vi "B-Lockin_time.vi"(7 "remote lockin address":string, 8 "error in (no error)":errorcluster, 9 "notifier":refnum<notifier>, 10 "Experiment Description":string="cool down\n\n", 11 "Experiment Folder":string="cooldown") -> (0 "error out":errorcluster)   [LabVIEW 2016, in "Transport.lvclass"]
uses:
  Transport.lvclass
  SweepControl/SweepControl.lvclass
  <userlib>/LevyLab/Levylab Instruments/Instrument Types/Cryostat/Instrument.Cryostat.lvclass
  <userlib>/LevyLab/LV to ITX/LVtoITX.lvclass
  Control Experiment/Control Experiment.lvclass
panel:
  in  "Tab Control":T1(tab)
  in  "milliseconds to wait":u32=1000
  in  "stop":bool
  out "X Channels":dbl[](array[numeric]) format="%#_6p"
  out "Y Channels":dbl[](array[numeric]) format="%#_6p"
  in  "append to existing file?\n(new file:F)":bool
  in  "Number of Channels to Save":i32=16
  in  "V2":i32=1 min=1
  in  "Current":i32=1 min=1
  in  "V1":i32=1 min=1
  out "Y":cluster{"Y":dbl[], "Y":dbl[]}[](graph)
  out "X":cluster{"Y":dbl[], "Y":dbl[]}[](graph)
  out "R vs time":cluster{"Y":dbl[], "Y":dbl[]}[](graph)
  out "Temperature vs time":cluster{"Y":dbl[], "Y":dbl[]}[](graph)
  out "R vs T":cluster{"Y":dbl[], "Y":dbl[]}[](graph)
  out "B vs Time":cluster{"Y":dbl[], "Y":dbl[]}[](graph)
  out "R vs B":cluster{"Y":dbl[], "Y":dbl[]}[](graph)
  in  "SweepControl.lvclass":refnum<class "SweepControl.lvclass">
  # "If V1 /= V2:\nR = (V1-V2)/I\nIf V1 = V2:\nR = V1/I"
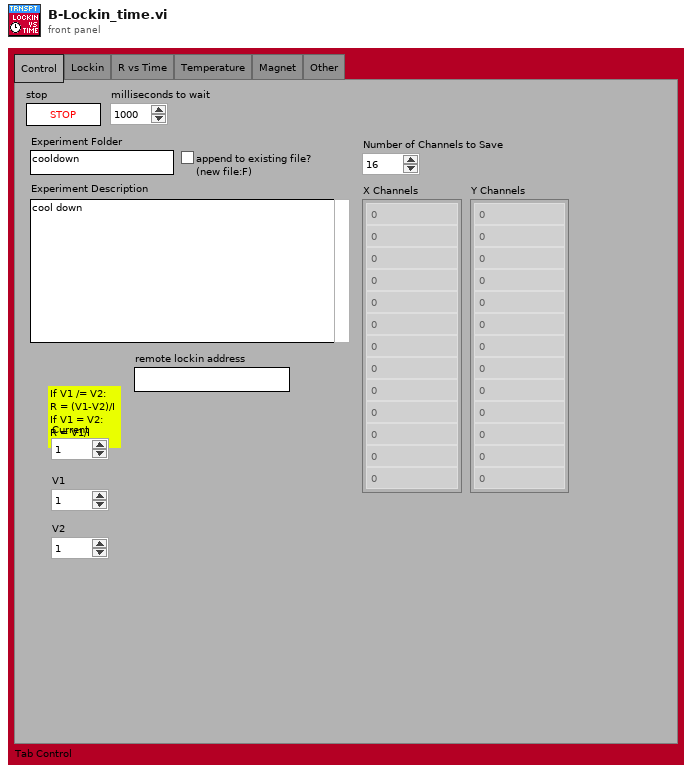
[diagram p1: front panel]
types:
  T1 = enum32{"Control", "Lockin", "R vs Time", "Temperature", "Magnet", "Other"}
  T2 = typedef "AO-cluster.ctl" = cluster{"AO amp (V)":T3, "AO DC (V)":T4, "AO f (Hz)":T5, "AO phi (°)":T6, "function":T7, "I+":bool[]}
  T3 = typedef "AO_Amp-array.ctl" = dbl[]
  T4 = typedef "AO_DC-array.ctl" = dbl[]
  T5 = typedef "AO_f-array.ctl" = dbl[]
  T6 = typedef "AO_phi-array.ctl" = dbl[]
  T7 = typedef "Function-array.ctl" = T8[]
  T8 = typedef "Function-enum.ctl" = enum16{"Sine", "Triangle", "Square", "Sawtooth"}
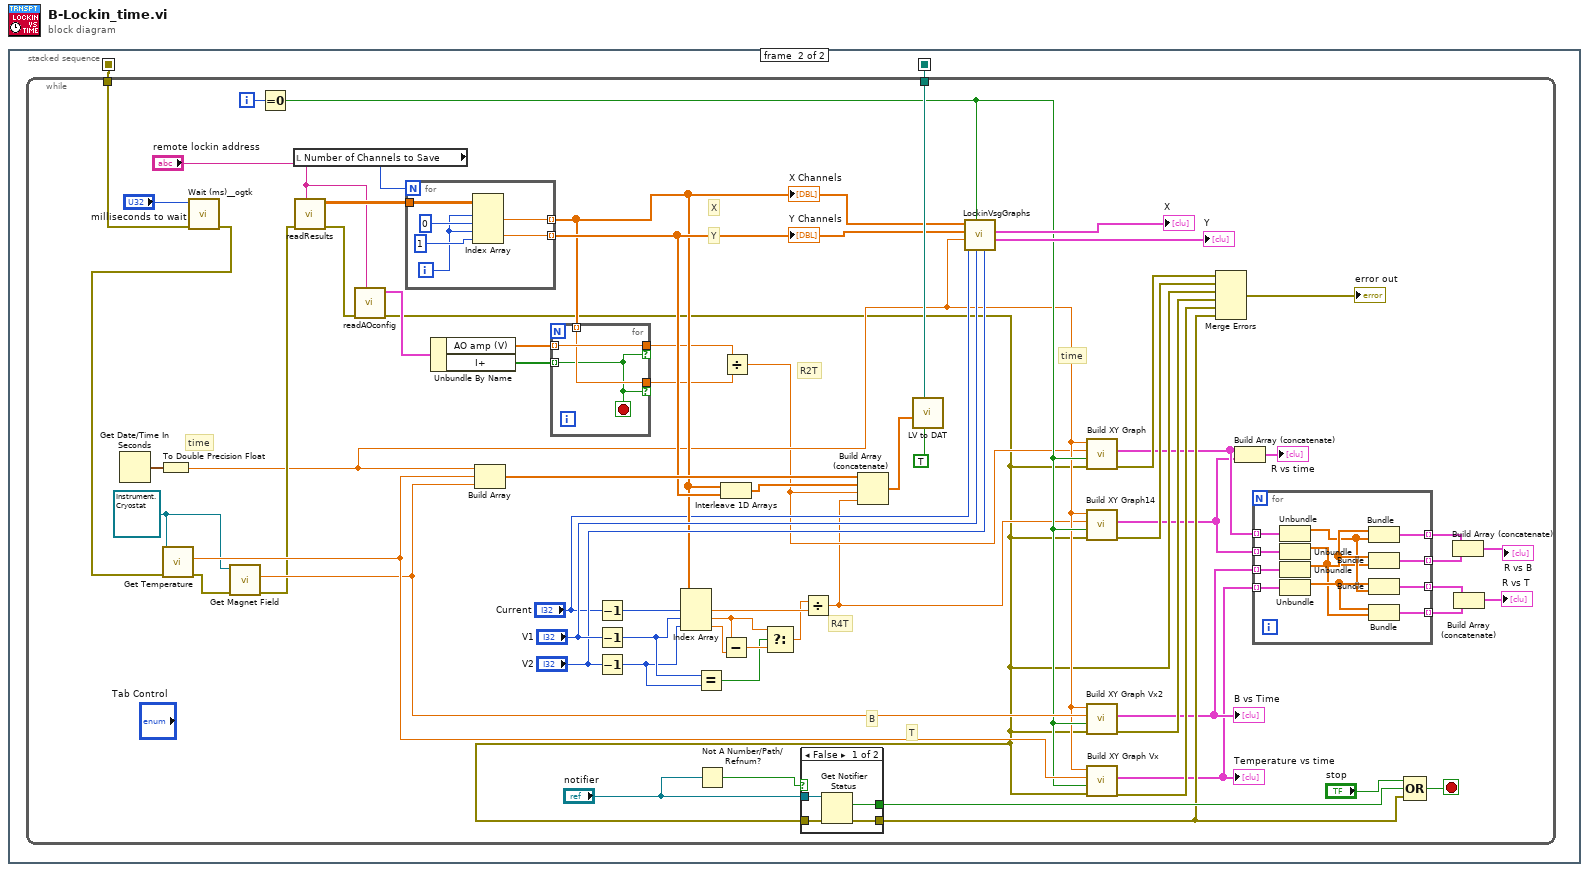
[diagram p0: block diagram]
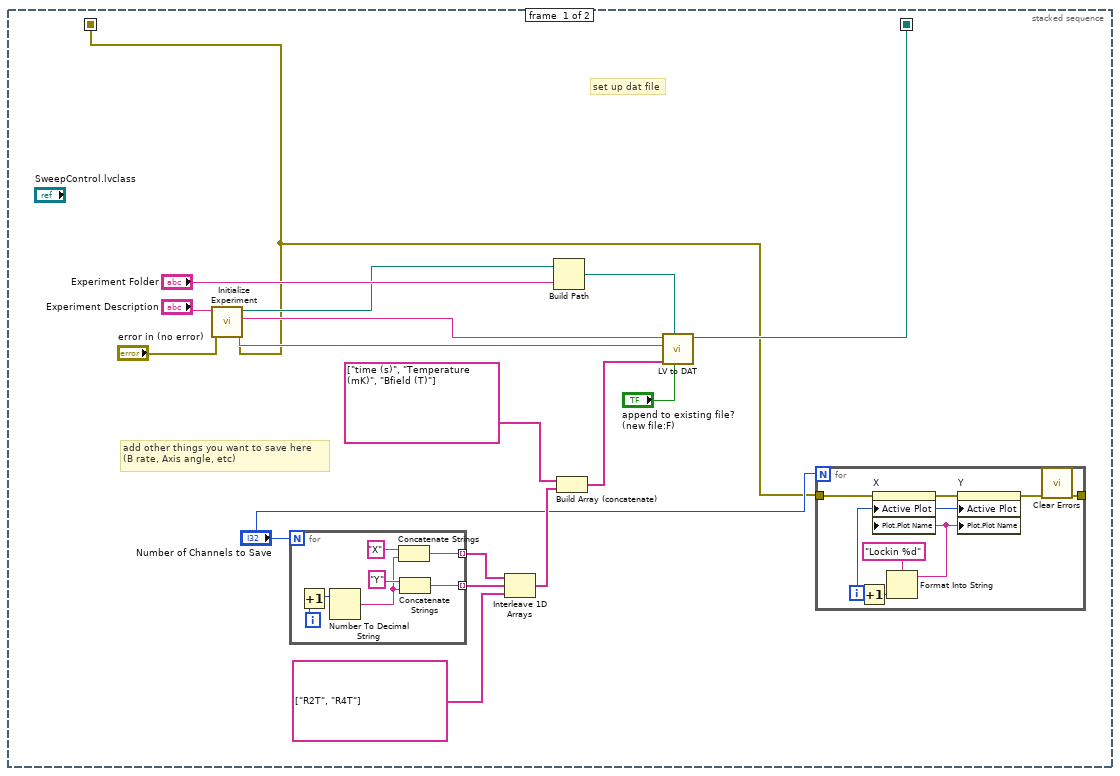
[diagram p2: hidden frame]
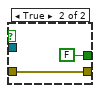
[diagram p3: hidden frame]
diagram:
  n1 = stacked-sequence {
    seq-local: [w3 _] -> [_ w34]
    seq-local: [w1 _] -> [_ w33]
    frame #0 {
      # "add other things you want to save here\n(B rate, Axis angle, etc)"
      # "set up dat file"
      n2 = call "Initialize Experiment.vi"("error in (no error)"="error in (no error)", "Experiment Comments"="Experiment Description") -> ("error out"=w1:errorcluster, "Comments"=w9:string, "device"=w8:string, "path"=w7:path)  [unwired: 6 in]
      n3 = for {
        N: "Number of Channels to Save" -> [_]
        tunnel: [w28] -> w13 mode=indexing
        tunnel: [w27] -> w12 mode=indexing
        i -> [w30]
        n4 = Increment(x=w30) -> (x+1=w26:i32)
        n5 = Number To Decimal String(number=w26) -> (decimal integer string=w29:string)  [unwired: 1 in]
        n6 = Concatenate Strings("X" ("wavenames"), w29) -> (w28:string)
        n7 = Concatenate Strings("Y" ("wavenames"), w29) -> (w27:string)
      }
      n8 = Interleave 1D Arrays(w13, w12, string[] ["R2T", "R4T"] ("wavenames (.Vx, etc)")) -> (w11:string[])
      n9 = Build Path(base path=w7, name or relative path="Experiment Folder") -> (appended path=w15:path)
      n10 = Build Array (concatenate)(string[] ["time (s)", "Temperature (mK)", "Bfield (T)"] ("wavenames (.Vx, etc)"), w11) -> (w14:string[])
      n11 = call <userlib>:"LV to DAT.vi"("append to file? (new file:F)"="append to existing file?\n(new file:F)", "path"=w15, "wavenames (.Vx, etc)"=w14, "Comments"=w9, "filename"=w8) -> ("new file path"=w3:path)  [unwired: 6 in]
      n12 = for {
        N: "Number of Channels to Save" -> [_]
        tunnel: [w24] -> _
        tunnel: w1 -> [w23]
        i -> [w21]
        n13 = Increment(x=w21) -> (x+1=w18:i32)
        n14 = Format Into String(format string="Lockin %d", w18) -> (resulting string=w22:string)  [unwired: 2 in, 1 out]
        n15 = property on="X" class="XYGraph (strict)"(error in=w23, "Active Plot"=w21, "Plot.Plot Name"=w22) -> (error out=w20:errorcluster)  [unwired: 1 in, 1 out]
        n16 = property on="Y" class="XYGraph (strict)"(error in=w20, "Active Plot"=w21, "Plot.Plot Name"=w22) -> (error out=w19:errorcluster)  [unwired: 1 in, 1 out]
        n17 = call <vilib>:"Clear Errors.vi"("error in (no error)"=w19) -> ("error out"=w24:errorcluster)  [unwired: 5 in, 1 out]
      }
    }
    frame #1 {
      n18 = while {
        tunnel: w34 -> [w100]
        tunnel: w33 -> [w78]
        i -> [w101]
        stop <- w70 stop-if-true
        w63 = refnum<class "Instrument.Cryostat.lvclass"> refnum ("Instrument.Cryostat in")
        # "R2T"
        # "R4T"
        # "T"
        # "B"
        # "time"
        # "Y"
        # "X"
        # "time"
        n19 = Get Date/Time In Seconds() -> (seconds since 1Jan1904=w98:timestamp)
        n20 = To Double Precision Float(number=w98) -> (double precision float=w50:dbl)
        n21 = call <userlib>:"Wait (ms)__ogtk.vi"("error in (no error)"=w78, "milliseconds to wait"="milliseconds to wait") -> ("error out"=w52:errorcluster)  [unwired: 8 in, 1 out]
        n22 = call-dynamic "Get Temperature.vi"("error in (no error)"=w52, "Instrument.Cryostat in"=w63) -> ("error out"=w65:errorcluster, "Temperature (K)"=w84:dbl)  [unwired: 6 in, 2 out]
        n23 = call-dynamic "Get Magnet Field.vi"("error in (no error)"=w65, "Instrument.Cryostat in"=w63) -> ("error out"=w64:errorcluster, "B Field (T)"=w79:dbl)  [unwired: 6 in, 2 out]
        n24 = Equal To 0?(x=w101) -> (x = 0?=w54:bool)
        n25 = local read "Number of Channels to Save"() -> (w93:i32)
        n26 = call <userlib>:"readResults.vi"("address"="remote lockin address", "error in (no error)"=w64) -> ("error out"=w62:errorcluster, "Results"=w99:dbl[][])  [unwired: 7 in, 1 out]
        n27 = call <userlib>:"readAOconfig.vi"("address"="remote lockin address", "error in (no error)"=w62) -> ("error out"=w46:errorcluster, "AOconfig"=w53:T2)  [unwired: 8 in]
        n28 = for {
          N: w93 -> [_]
          tunnel: w99 -> [w126]
          tunnel: [w124] -> w59 mode=indexing
          tunnel: [w125] -> w66 mode=indexing
          i -> [w123]
          n29 = Index Array(array=w126, index (row) #1=w123, index (col) #1=0 ("disabled index (col)"), index (row) #2=w123, index (col) #2=1 ("disabled index (col)")) -> (element #1=w124:dbl, element #2=w125:dbl)
        }
        "X Channels" <- w59
        "Y Channels" <- w66
        n30 = Unbundle By Name(w53) -> ("AO amp (V)"=w61:T3, "I+"=w60:bool[])
        n31 = Build Array(w50, w84, w79) -> (w94:dbl[])
        n32 = for {
          tunnel: w61 -> [w116] mode=indexing
          tunnel: w60 -> [w114] mode=indexing
          tunnel: [w116] -> w58 if=w114
          tunnel: [w115] -> w57 if=w114
          tunnel: w59 -> [w115] mode=indexing
          stop <- w114 stop-if-true
        }
        n33 = Decrement(x="Current") -> (x-1=w92:i32)
        n34 = Decrement(x="V1") -> (x-1=w88:i32)
        n35 = Decrement(x="V2") -> (x-1=w87:i32)
        n36 = Index Array(array=w59, index #1=w92, index #2=w88, index #3=w87) -> (element #1=w96:dbl, element #2=w89:dbl, element #3=w91:dbl)
        n37 = Equal?(x=w88, y=w87) -> (x = y?=w86:bool)
        n38 = Not A Number/Path/Refnum?(number/path/refnum="notifier") -> (NaN/Path/Refnum?=w67:bool)
        n39 = Interleave 1D Arrays(w59, w66) -> (w56:dbl[])
        n40 = Subtract(x=w89, y=w91) -> (x-y=w90:dbl)
        n41 = Divide(x=w58, y=w57) -> (x/y=w49:dbl)
        n42 = Select(t=w89, s=w86, f=w90) -> (s? t:f=w85:dbl)
        n43 = case shown="False" w67 {
          tunnel: [w120 FALSE] -> w71
          tunnel: [w119 w121] -> w69
          tunnel: "notifier" -> [w118 _]
          tunnel: w46 -> [w117 w121]
          frame False {
            n44 = Get Notifier Status(notifier=w118, error in (no error)=w117) -> (current notification=w120:bool, error out=w119:errorcluster)  [unwired: 3 out]
          }
          frame True {
          }
        }
        n45 = Divide(x=w85, y=w96) -> (x/y=w47:dbl)
        n46 = Build Array (concatenate)(w94, w56, w49, w47) -> (w51:dbl[])
        n47 = call <userlib>:"LV to DAT.vi"("append to file? (new file:F)"=TRUE, "path"=w100, "Data"=w51) -> ()  [unwired: 8 in, 1 out]
        n48 = call "LockinVsgGraphs.vi"("V2"="V2", "V1"="V1", "reset?"=w54, "Current"="Current", "parameter in"=w50, "Y array in"=w66, "X array in"=w59) -> ("Y vs Parameter"=→"Y":cluster{"Y":dbl[], "Y":dbl[]}[], "X vs Parameter"=→"X":cluster{"Y":dbl[], "Y":dbl[]}[])  [unwired: 2 in, 1 out]
        n49 = call "Build XY Graph"("error in (no error)"=w46, "Reset"=w54, "Y Input"=w49, "X Input"=w50) -> ("error out"=w77:errorcluster, "XY Graph"=w45:cluster{"Y":dbl[], "Y":dbl[]}[])  [unwired: 1 in, 5 out]
        n50 = call "Build XY Graph14"("error in (no error)"=w46, "Reset"=w54, "Y Input"=w47, "X Input"=w50) -> ("error out"=w76:errorcluster, "XY Graph"=w44:cluster{"Y":dbl[], "Y":dbl[]}[])  [unwired: 1 in, 5 out]
        n51 = call "Build XY Graph Vx2"("error in (no error)"=w46, "Reset"=w54, "Y Input"=w79, "X Input"=w50) -> ("error out"=w75:errorcluster, "XY Graph"=w43:cluster{"Y":dbl[], "Y":dbl[]}[])  [unwired: 1 in, 5 out]
        "B vs Time" <- w43
        n52 = call "Build XY Graph Vx"("error in (no error)"=w46, "Reset"=w54, "Y Input"=w84, "X Input"=w50) -> ("error out"=w74:errorcluster, "XY Graph"=w42:cluster{"Y":dbl[], "Y":dbl[]}[])  [unwired: 1 in, 5 out]
        "Temperature vs time" <- w42
        n53 = Merge Errors(w77, w76, w46, w75, w74, w69) -> (→"error out":errorcluster)
        n54 = Build Array (concatenate)(w45, w44) -> (→"R vs time":cluster{"Y":dbl[], "Y":dbl[]}[])
        n55 = for {
          tunnel: w45 -> [w113] mode=indexing
          tunnel: w44 -> [w112] mode=indexing
          tunnel: w43 -> [w111] mode=indexing
          tunnel: w42 -> [w110] mode=indexing
          tunnel: [w105] -> w41 mode=indexing
          tunnel: [w104] -> w40 mode=indexing
          tunnel: [w103] -> w38 mode=indexing
          tunnel: [w102] -> w37 mode=indexing
          n56 = Unbundle(w113) -> ("Y"=w107:dbl[])  [unwired: 1 out]
          n57 = Unbundle(w112) -> ("Y"=w106:dbl[])  [unwired: 1 out]
          n58 = Unbundle(w111) -> ("Y"=w108:dbl[])  [unwired: 1 out]
          n59 = Unbundle(w110) -> ("Y"=w109:dbl[])  [unwired: 1 out]
          n60 = Bundle("Y"=w108, "Y"=w107) -> (w105:cluster{"Y":dbl[], "Y":dbl[]})  [unwired: 1 in]
          n61 = Bundle("Y"=w108, "Y"=w106) -> (w104:cluster{"Y":dbl[], "Y":dbl[]})  [unwired: 1 in]
          n62 = Bundle("Y"=w109, "Y"=w107) -> (w103:cluster{"Y":dbl[], "Y":dbl[]})  [unwired: 1 in]
          n63 = Bundle("Y"=w109, "Y"=w106) -> (w102:cluster{"Y":dbl[], "Y":dbl[]})  [unwired: 1 in]
        }
        n64 = Compound Arithmetic op=OR("stop", w71, w69) -> (w70:bool)
        n65 = Build Array (concatenate)(w41, w40) -> (→"R vs B":cluster{"Y":dbl[], "Y":dbl[]}[])
        n66 = Build Array (concatenate)(w38, w37) -> (→"R vs T":cluster{"Y":dbl[], "Y":dbl[]}[])
      }
    }
  }
